vi "MCP23S17 Read.vi"(7 "error in (no error)":errorcluster, 9 "Addr":T1 items=["Addr-0"=0, "Addr-1"=4, "Addr-2"=2, "Addr-3"=6, "Addr-4"=1, "Addr-5"=5, "Addr-6"=3, "Addr-7"=7], 10 "handle":u32 format="%08x") -> (0 "error out":errorcluster, 1 "REG B":u16, 2 "REG A":u16, 3 "handle out":u32, 4 "Str out B":string, 6 "Str out A":string)   [LabVIEW 2018]
uses:
  PROJEKT/NIKO/Labview/Niko V4/FTDI SPI/Ctl/Sub Addr.ctl
  PROJEKT/NIKO/Labview/Niko V6_A/FTDI SPI/libMPSSE-SPI.lvlib
panel:
  out "string":string
  in  "Array U8":u8[](array[numeric])=[64, 18, 0, 128, 0, 0, 0, 0, 0, 0] format="%x"
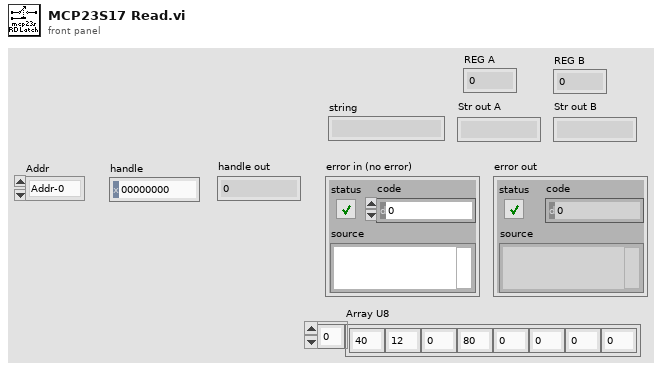
[diagram p1: front panel]
types:
  T1 = typedef "Sub Addr.ctl" = u16
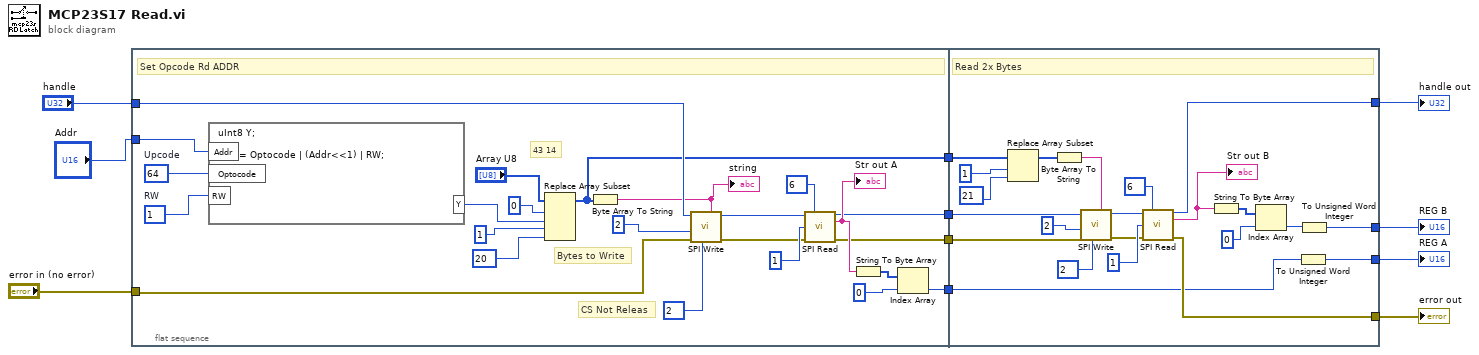
[diagram p0: block diagram]
diagram:
  n1 = flat-sequence {
    tunnel: "Addr" -> [w34]
    tunnel: "handle" -> [w30]
    tunnel: "error in (no error)" -> [w27]
    tunnel: [w15] -> w8
    tunnel: [w14] -> w7
    tunnel: [w13] -> w6
    tunnel: [w12] -> w5
    tunnel: [w55] -> w9
    tunnel: [w54] -> w4
    tunnel: w8 -> [w49]
    tunnel: w7 -> [w45]
    tunnel: w6 -> [w43]
    tunnel: w5 -> [w38]
    tunnel: [w37] -> w2
    tunnel: [w36] -> w1
    frame #0 {
      w23 = u8 64  # Upcode
      w24 = u8 1  # RW
      # "CS Not Releas"
      # "Bytes to Write"
      # "43 14"
      # "Set Opcode Rd ADDR"
      n2 = formula code="uInt8 Y;\n      \n    Y = Optocode | (Addr<<1) | RW;"("Addr"=w34, "Optocode"=w23, "RW"=w24) -> ("Y"=w33:u8)
      n3 = Replace Array Subset(array="Array U8", new element #1=w33, index #1=0 ("index"), new element #2=u8 20, index #2=u8 1 ("new element/subarray")) -> (w15:u8[])
      n4 = Byte Array To String(unsigned byte array=w15) -> (string=w29:string)
      "string" <- w29
      n5 = call "SPI Write.vi"("buffer"=w29, "options"=u8 2, "error in (no error)"=w27, "Bytes To Send"=u32 2, "handle"=w30) -> ("error out"=w19:errorcluster, "handle out"=w20:u32)  [unwired: 4 in, 1 out]
      n6 = call "SPI Read.vi"("handle"=w20, "options"=u8 6, "sizeToTransfer"=u32 1, "error in (no error)"=w19) -> ("handle out"=w14:u32, "buffer out"=w16:string, "error out"=w13:errorcluster)  [unwired: 7 in, 2 out]
      "Str out A" <- w16
      n7 = String To Byte Array(string=w16) -> (unsigned byte array=w17:u8[])
      n8 = Index Array(array=w17, index=0) -> (element=w12:u8)
    }
    frame #1 {
      # "Read 2x Bytes"
      n9 = Replace Array Subset(array=w49, new element=u8 21, index=u8 1 ("new element/subarray")) -> (w46:u8[])
      n10 = Byte Array To String(unsigned byte array=w46) -> (string=w44:string)
      n11 = call "SPI Write.vi"("buffer"=w44, "options"=u8 2, "error in (no error)"=w43, "Bytes To Send"=u32 2, "handle"=w45) -> ("error out"=w42:errorcluster, "handle out"=w41:u32)  [unwired: 4 in, 1 out]
      n12 = call "SPI Read.vi"("handle"=w41, "options"=u8 6, "sizeToTransfer"=u32 1, "error in (no error)"=w42) -> ("handle out"=w54:u32, "buffer out"=w53:string, "error out"=w55:errorcluster)  [unwired: 7 in, 2 out]
      "Str out B" <- w53
      n13 = String To Byte Array(string=w53) -> (unsigned byte array=w52:u8[])
      n14 = Index Array(array=w52, index=0) -> (element=w50:u8)
      n15 = To Unsigned Word Integer(number=w38) -> (unsigned 16bit integer=w36:u16)
      n16 = To Unsigned Word Integer(number=w50) -> (unsigned 16bit integer=w37:u16)
    }
  }
  "error out" <- w9
  "handle out" <- w4
  "REG B" <- w2
  "REG A" <- w1
